vi "binsert.vi"(10 "String":string, 11 "strings":string[](array[string])) -> (3 "index":i32)   [LabVIEW 2013]
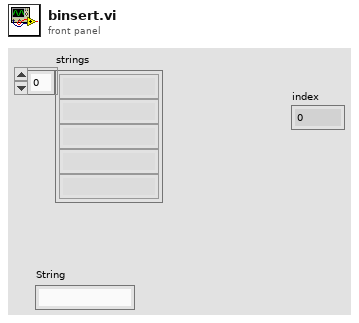
[diagram p1: front panel]
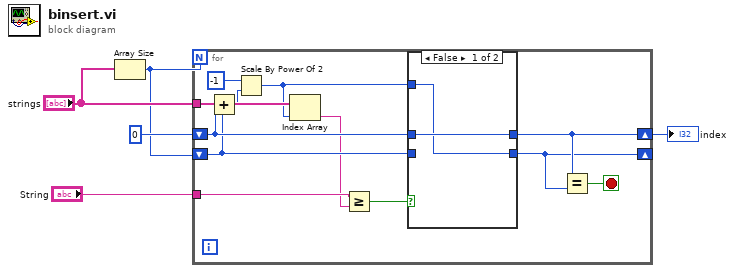
[diagram p0: block diagram]
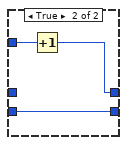
[diagram p2: hidden frame]
diagram:
  n1 = Array Size(array="strings") -> (size(s)=w2:i32)
  n2 = for {
    N: w2 -> [_]
    tunnel: "strings" -> [w17]
    tunnel: "String" -> [w11]
    shift-right: [w7] -> _
    shift-left: w2 -> [w12]
    shift-right: [w8] -> w1
    shift-left: 0 -> [w13]
    stop <- w6 stop-if-true
    n3 = Add(x=w13, y=w12) -> (x+y=w15:i32)
    n4 = Scale By Power Of 2(n=i16 -1, x=w15) -> (x*2^n=w14:i32)
    n5 = Index Array(array=w17, index=w14) -> (element=w10:string)
    n6 = Greater Or Equal?(x=w11, y=w10) -> (x >= y?=w9:bool)
    n7 = case shown="False" w9 {
      tunnel: w14 -> [w18 w22]
      tunnel: [w18 w20] -> w7
      tunnel: w13 -> [w19 _]
      tunnel: [w19 w21] -> w8
      tunnel: w12 -> [_ w20]
      frame False {
      }
      frame True {
        n8 = Increment(x=w22) -> (x+1=w21:i32)
      }
    }
    n9 = Equal?(x=w8, y=w7) -> (x = y?=w6:bool)
  }
  "index" <- w1
